vi "FindBow.vi"(11 "Refnum in":T3) -> (0 "Bow Heading":T2 format="%05.1f", 1 "Bow found?":T1, 2 "bow pixel y":i32, 3 "bow pixel x":i32)   [LabVIEW 2011]
uses:
  <vilib>/vision/Image Controls.llb/IMAQ Image.ctl
  2-RIO/2 Typedefs/heading.ctl
  2-RIO/2 Typedefs/indicator LED.ctl
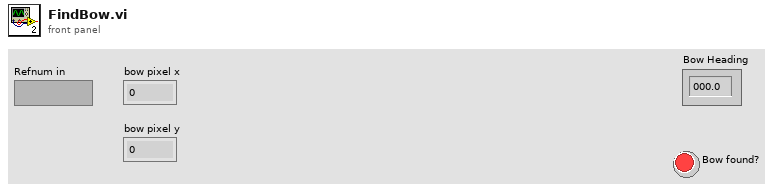
[diagram p1: front panel]
types:
  T1 = typedef "indicator LED.ctl" = bool
  T2 = typedef "heading.ctl" = dbl
  T3 = typedef "IMAQ Image.ctl" = refnum<image>
  T4 = cluster{"Position":cluster{"x":sgl, "y":sgl}, "Angle":sgl, "Scale":sgl, "Score":sgl, "Bounding Box":cluster{"x":sgl, "y":sgl}[]}[]
  T5 = cluster{"Position":cluster{"x":sgl, "y":sgl}, "Angle":sgl, "Scale":sgl, "Score":sgl, "Bounding Box":cluster{"x":sgl, "y":sgl}[]}
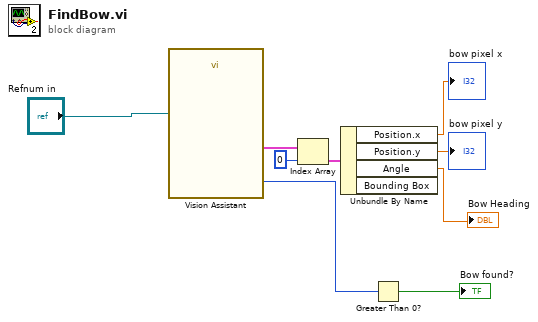
[diagram p0: block diagram]
diagram:
  n1 = call "Vision Assistant"("Image In"="Refnum in") -> ("Matches (Color Pattern Matching 1)"=w6:T4, "Number of Matches (Color Pattern Matching 1)"=w3:i32)  [unwired: 23 in, 2 out]
  n2 = Index Array(array=w6, index=0) -> (element=w5:T5)
  n3 = Unbundle By Name(w5) -> ("Position.x"=→"bow pixel x":sgl, "Position.y"=→"bow pixel y":sgl, "Angle"=→"Bow Heading":sgl)  [unwired: 1 out]
  n4 = Greater Than 0?(x=w3) -> (x > 0?=→"Bow found?":bool)
